vi "MazeEdgeTracking.vi"(10 "Refnum in":T1, 11 "Refnum in":T2) -> (0 "output cluster 2":cluster{"Numeric 2":sgl, "Numeric":sgl}, 1 "output cluster":cluster{"Numeric 2":sgl, "Numeric":sgl}, 3 "Refnum out":T1)   [LabVIEW 2021]
uses:
  <vilib>/vision/Image Controls.llb/IMAQ Image.ctl
  <vilib>/userDefined/High Color/IMAQdx.ctl
  <vilib>/vision/driver/IMAQdx.llb/IMAQdx Buffer Number Mode.ctl
  <vilib>/vision/Management.llb/Cast Image 2 Method.ctl
  <vilib>/vision/Shape Detection.llb/ShapeDetectionMatchOptions.ctl
  <vilib>/vision/Pattern Matching.llb/IMAQ Match Range Setting.ctl
  <vilib>/vision/driver/NI_Vision_Acquisition_Software.lvlib
  <vilib>/vision/NI_Vision_Development_Module.lvlib
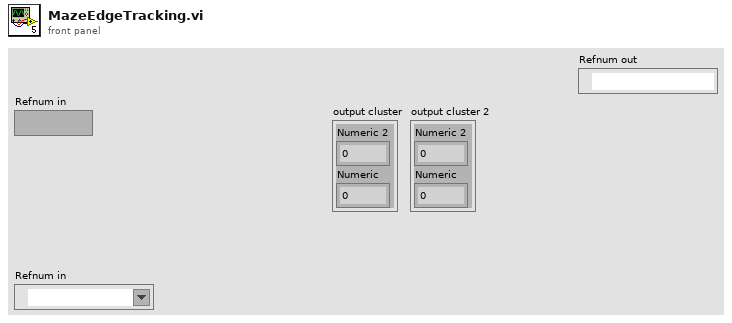
[diagram p1: front panel]
types:
  T1 = typedef "IMAQdx.ctl" = refnum<k21>
  T2 = typedef "IMAQ Image.ctl" = refnum<image>
  T3 = cluster{"Min Width":dbl, "Max Width":dbl, "Min Height":dbl, "Max Height":dbl}
  T4 = typedef "ShapeDetectionMatchOptions.ctl" = cluster{"Rotation":bool, "Scale":bool, "Occlusion":bool, "Range Settings":T5[]}
  T5 = typedef "IMAQ Match Range Setting.ctl" = cluster{"Match Constraints":u32, "Min":dbl, "Max":dbl}
  T6 = typedef "IMAQ Rectangle" = cluster{"Left":i32, "Top":i32, "Right":i32, "Bottom":i32, "Rotation":dbl}
  T7 = typedef "Cast Image 2 Method.ctl" = u32
  T8 = typedef "Image Type" = u32
  T9 = typedef "NI_Vision_Acquisition_Software.lvlib/IMAQdx Buffer Number Mode.ctl" = enum32{"Next", "Last", "Buffer Number", "Every", "Last New"}
  T10 = typedef "ROI Descriptor" = cluster{"Global Rectangle":i32[], "Contours":cluster{"ID":enum32{"External", "Internal"}, "Type":u32, "Coordinates":i32[]}[]}
  T11 = cluster{"Corners":cluster{"X":sgl, "Y":sgl}[], "Angle":dbl, "Width":dbl, "Height":dbl, "Score":dbl}[]
  T12 = cluster{"Corners":cluster{"X":sgl, "Y":sgl}[], "Angle":dbl, "Width":dbl, "Height":dbl, "Score":dbl}
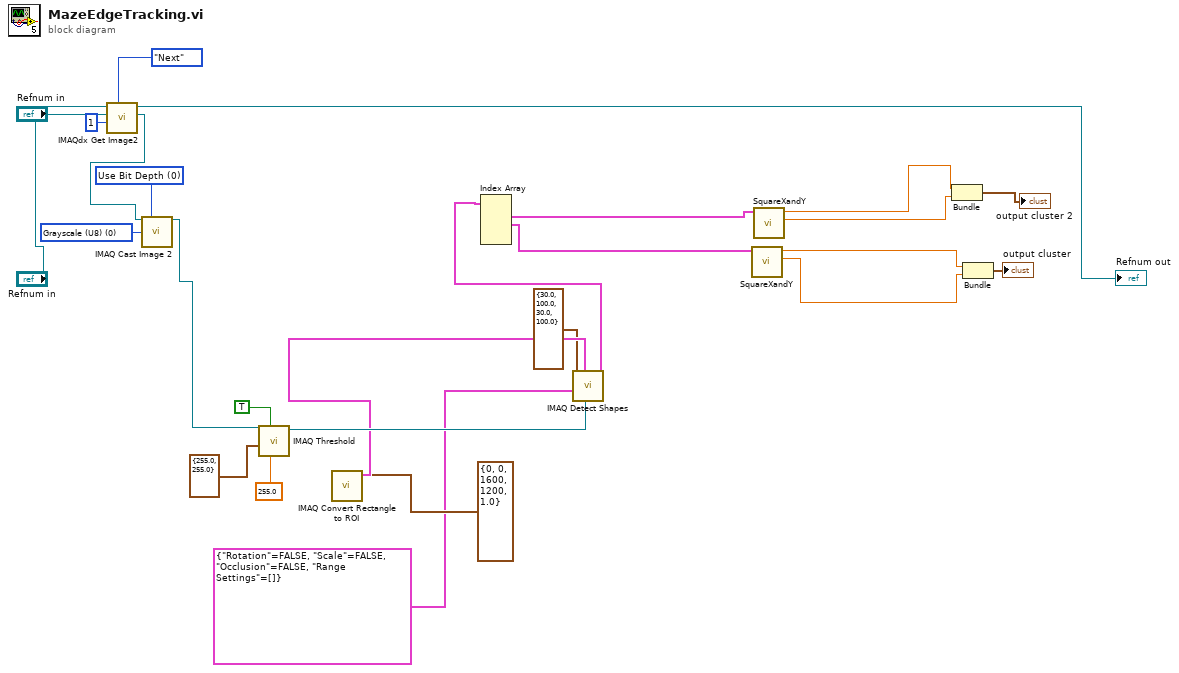
[diagram p0: block diagram]
diagram:
  w15 = T7 0 items=["Use Bit Depth", "Shift", "Use Lookup Table"] ("Method")
  w14 = T8 0 items=["Grayscale (U8)", "Grayscale (I16)", "Grayscale (SGL)", "Complex (CSG)", "RGB (U32)", "HSL (U32)", "RGB (U64)", "Grayscale (U16)"] ("Image Type")
  n1 = call <vilib>:"IMAQdx Get Image2.vi"("Buffer Number Mode (Next)"=IMAQdx_Buffer_Number_Mode."Next", "Buffer Number In"=u32 1, "Image In"="Refnum in", "Session In"="Refnum in") -> ("Image Out"=w26:T2, "Session Out"=→"Refnum out":T1)  [unwired: 4 in, 2 out]
  n2 = call "IMAQ Cast Image 2"("Image Src"=w26, "Method"=w15, "Image Type"=w14) -> ("Image Dst Out"=w16:T2)  [unwired: 11 in, 1 out]
  n3 = call "IMAQ Threshold"("Replace Value"=sgl 255.0, "Keep/Replace Value (Replace)"=TRUE, "Range"=cluster{"Upper value":sgl, "Lower value":sgl} {"Upper value"=255.0, "Lower value"=255.0}, "Image Src"=w16) -> ("Image Dst Out"=w20:T2)  [unwired: 6 in, 1 out]
  n4 = call "IMAQ Convert Rectangle to ROI"("Rectangle"=T6 {"Left"=0, "Top"=0, "Right"=1600, "Bottom"=1200, "Rotation"=1.0}) -> ("ROI Descriptor"=w19:T10)  [unwired: 8 in, 1 out]
  n5 = call-poly "IMAQ Detect Shapes"("ROI Descriptor"=w19, "Match Options"=T4 {"Rotation"=FALSE, "Scale"=FALSE, "Occlusion"=FALSE, "Range Settings"=[]}, "Rectangle Descriptor"=T3 {"Min Width"=30.0, "Max Width"=100.0, "Min Height"=30.0, "Max Height"=100.0}, "Image"=w20) -> ("Rectangles"=w25:T11)  [unwired: 5 in, 2 out]
  n6 = Index Array(array=w25) -> (element #1=w9:T12, element #2=w8:T12)  [unwired: 4 in, 2 out]
  n7 = call "SquareXandY.vi"("Rectangle Descriptor"=w8) -> ("Numeric"=w4:sgl, "Numeric 2"=w5:sgl)  [unwired: 9 in]
  n8 = call "SquareXandY.vi"("Rectangle Descriptor"=w9) -> ("Numeric"=w6:sgl, "Numeric 2"=w7:sgl)  [unwired: 9 in]
  n9 = Bundle("Numeric 2"=w7, "Numeric"=w6) -> (→"output cluster 2":cluster{"Numeric 2":sgl, "Numeric":sgl})  [unwired: 1 in]
  n10 = Bundle("Numeric 2"=w5, "Numeric"=w4) -> (→"output cluster":cluster{"Numeric 2":sgl, "Numeric":sgl})  [unwired: 1 in]
